vi "流量计UI.vi"() -> ()   [LabVIEW 2016, in "流量计集成.lvlib"]
uses:
  <vilib>/Utility/miscctls.llb/LVPointTypeDef.ctl
  SL1500-3G/SL1500-3G.lvlib
panel:
  in  "返回":bool
  in  "设置":bool
  in  "流量计类型":T1
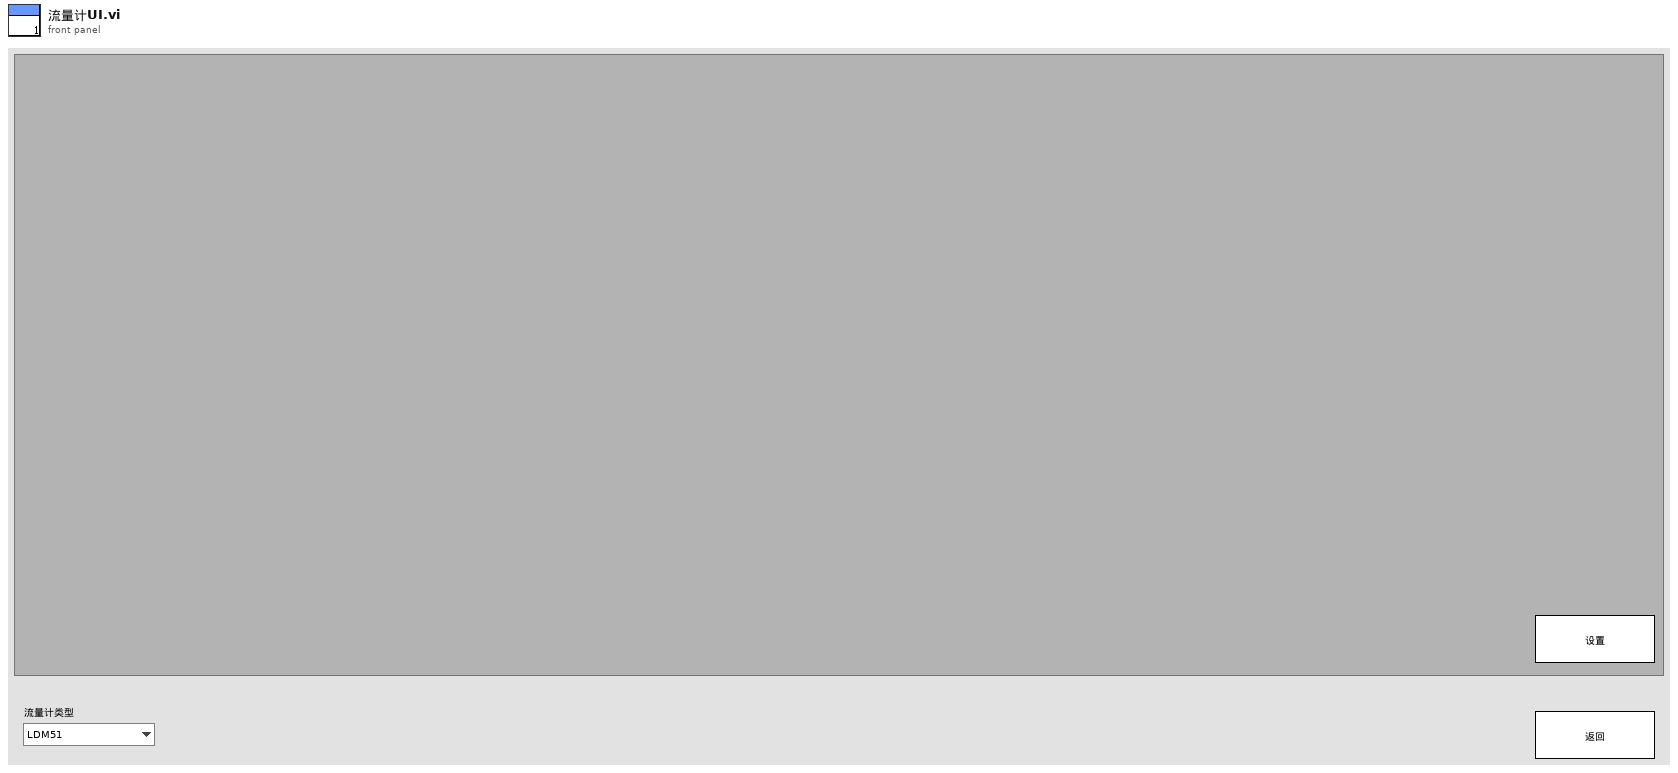
[diagram p1: front panel]
types:
  T1 = typedef "流量计集成.lvlib/流量计类型.ctl" = enum16{"LDM51", "MGG/KL QC", "斯坦道功率测流", "LSH10-1QC流量计", "SL1500-3G", "WL1A1明渠流量计", "LSS-100X流量计"}
  T2 = typedef "LVPointTypeDef.ctl" = cluster{"Horizontal":i16, "Vertical":i16}
  T3 = enum32{"Bad", "Idle", "Run top level", "Running"}
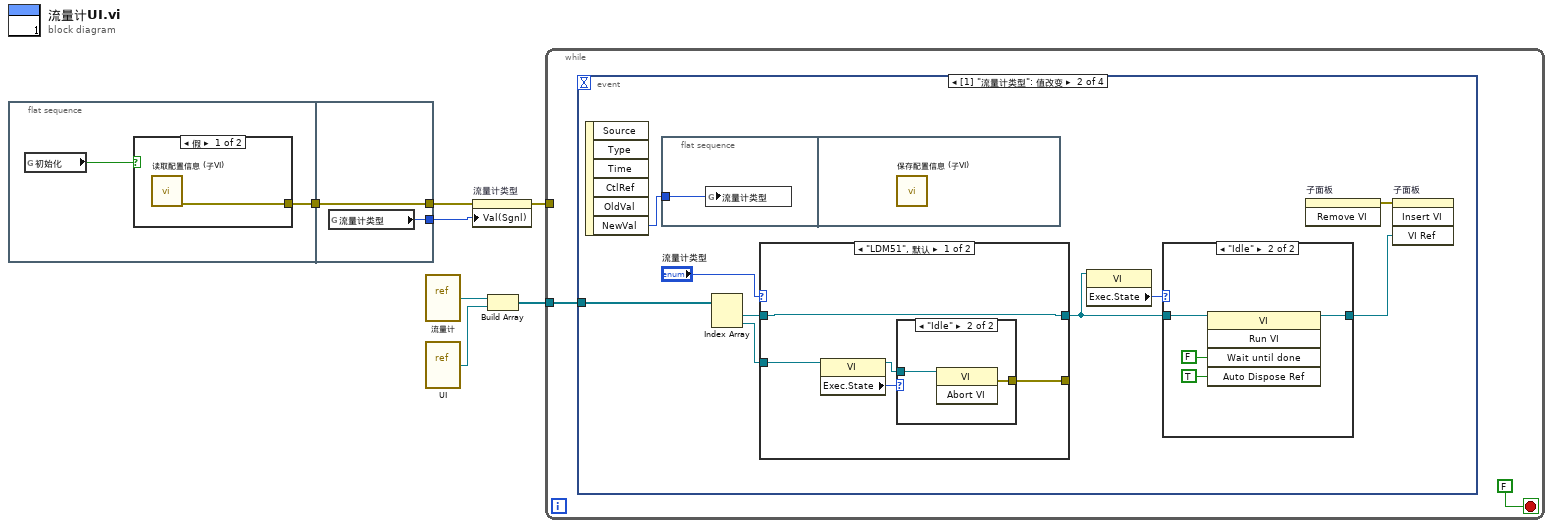
[diagram p0: block diagram]
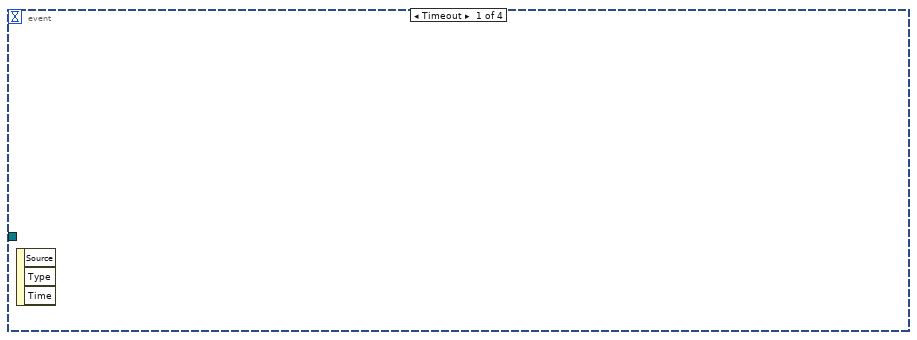
[diagram p3: hidden frame]
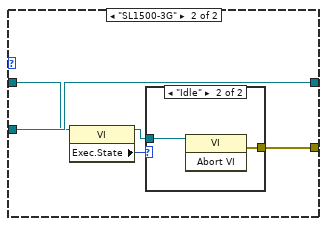
[diagram p6: hidden frame]
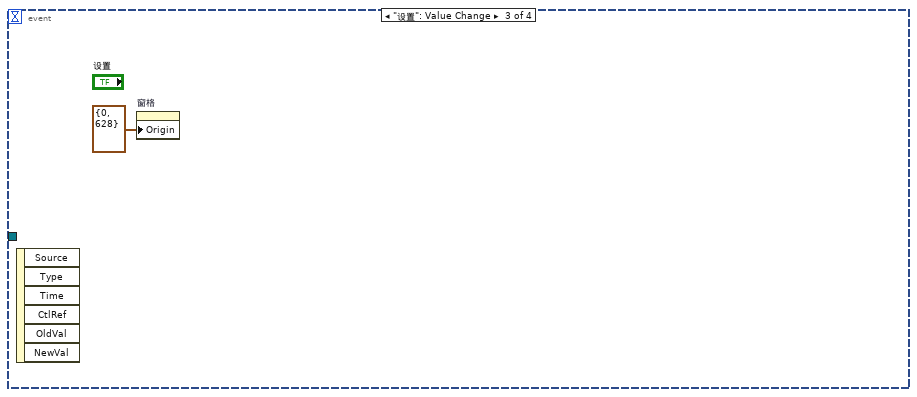
[diagram p8: hidden frame]
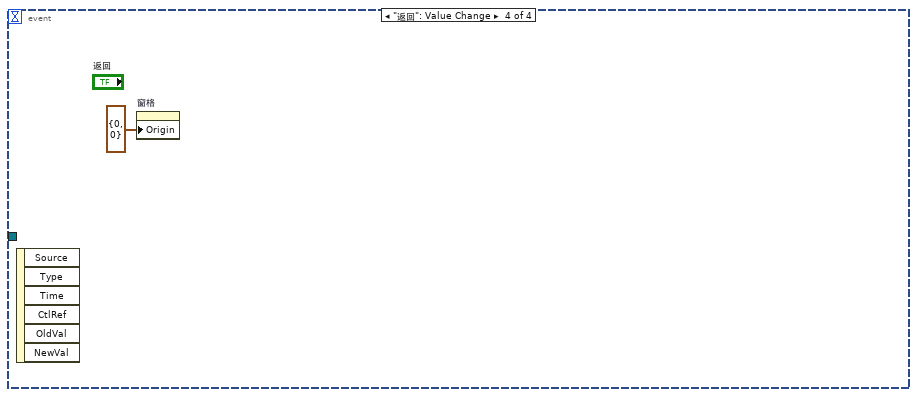
[diagram p9: hidden frame]
diagram:
  n1 = flat-sequence {
    tunnel: [w9] -> w3
    tunnel: w3 -> [w11]
    tunnel: [w12] -> w2
    tunnel: [w11] -> w1
    frame #0 {
      n2 = global read "流量计全局变量.vi" "初始化"() -> (w8:bool)
      n3 = case shown="假" w8 {
        tunnel: [w10 _] -> w9
        frame False {
          n4 = call "读取配置信息 (子VI).vi"() -> ("错误输出"=w10:errorcluster)  [unwired: 11 in]
        }
        frame True {
        }
      }
    }
    frame #1 {
      n5 = global read "流量计全局变量.vi" "流量计类型"() -> (w12:T1)
    }
  }
  n6 = vi-ref "流量计.vi"() -> (w7:refnum<vi>)
  n7 = vi-ref "UI.vi"() -> (w6:refnum<vi>)
  n8 = property on="流量计类型" class="Enum (严格)"(error in=w1, "Val(Sgnl)"=w2) -> (error out=w4:errorcluster)  [unwired: 1 in, 1 out]
  n9 = Build Array(w7, w6) -> (w5:refnum<vi>[])
  n10 = while {
    tunnel: w5 -> [w13]
    tunnel: w4 -> [_]
    stop <- FALSE stop-if-true
    n11 = event shown="[1] \"流量计类型\": 值改变" {
      selector: _ -> [_ _ _ _]
      dyn-events: _ -> [_ _ _ _]
      timeout: _ -> [_ _ _ _]
      tunnel: w13 -> [_ w20 _ _]
      event Timeout {
        n12 = event-data() -> ()  [unwired: 1 in, 3 out]
      }
      event Value Change {
        n13 = event-data() -> ("NewVal"=w15:T1)  [unwired: 1 in, 5 out]
        n14 = flat-sequence {
          tunnel: w15 -> [w24]
          frame #0 {
            n15 = global write "流量计全局变量.vi" "流量计类型"(w24) -> ()
          }
          frame #1 {
            n16 = call "保存配置信息 (子VI).vi"() -> ()  [unwired: 11 in, 1 out]
          }
        }
        n17 = Index Array(array=w20) -> (element #1=w19:refnum<vi>, element #2=w18:refnum<vi>)  [unwired: 2 in]
        n18 = case shown="\"LDM51\", 默认" "流量计类型" {
          tunnel: [w34 w41] -> w17
          tunnel: w19 -> [w34 w40]
          tunnel: w18 -> [w33 w41]
          tunnel: [w32 w39] -> _
          frame "LDM51", Default {
            n19 = property class="VI"(reference=w33) -> (reference out=w31:refnum<vi>, "Exec.State"=w30:T3)  [unwired: 1 in, 1 out]
            n20 = case shown="\"Idle\"" w30 {
              tunnel: [_ w36] -> w32
              tunnel: w31 -> [_ w35]
              frame "Bad", Default {
              }
              frame "Idle" {
                n21 = invoke class="VI" method="Abort VI"(reference=w35) -> (error out=w36:errorcluster)  [unwired: 2 in, 2 out]
              }
            }
          }
          frame "SL1500-3G" {
            n22 = property class="VI"(reference=w40) -> (reference out=w38:refnum<vi>, "Exec.State"=w37:T3)  [unwired: 1 in, 1 out]
            n23 = case shown="\"Idle\"" w37 {
              tunnel: [_ w43] -> w39
              tunnel: w38 -> [_ w42]
              frame "Bad", Default {
              }
              frame "Idle" {
                n24 = invoke class="VI" method="Abort VI"(reference=w42) -> (error out=w43:errorcluster)  [unwired: 2 in, 2 out]
              }
            }
          }
        }
        n25 = property class="VI"(reference=w17) -> ("Exec.State"=w16:T3)  [unwired: 1 in, 2 out]
        n26 = case shown="\"Idle\"" w16 {
          tunnel: [w25 w29] -> w22
          tunnel: w17 -> [w25 w26]
          frame "Bad", Default {
          }
          frame "Idle" {
            n27 = invoke class="VI" method="Run VI"(reference=w26, "Wait until done"=FALSE ("结束前等待"), "Auto Dispose Ref"=TRUE ("自动销毁引用")) -> (reference out=w29:refnum<vi>)  [unwired: 2 in, 4 out]
          }
        }
        n28 = invoke on="子面板" class="SubPnl" method="Remove VI"() -> (error out=w23:errorcluster)  [unwired: 3 in, 2 out]
        n29 = invoke on="子面板" class="SubPnl" method="Insert VI"(error in=w23, "VI Ref"=w22) -> ()  [unwired: 2 in, 4 out]
      }
      event "设置": Value Change {
        n30 = event-data() -> ()  [unwired: 1 in, 6 out]
        n31 = property on="窗格" class="Pane"("Origin"=T2 {"Horizontal"=0, "Vertical"=628} ("原点")) -> ()  [unwired: 2 in, 2 out]
      }
      event "返回": Value Change {
        n32 = event-data() -> ()  [unwired: 1 in, 6 out]
        n33 = property on="窗格" class="Pane"("Origin"=T2 {"Horizontal"=0, "Vertical"=0} ("原点")) -> ()  [unwired: 2 in, 2 out]
      }
    }
  }
